vi "tb_Ping Pong BRAM.vi"() -> ()   [LabVIEW 2011]
panel:
  out "interleaved array":dbl[](array[numeric])
  out "Array 2":u16[](array[numeric])
  out "Array":u16[](array[numeric])
  out "Memory":u16[](array[numeric])
  in  "Iterations":i32=100
  out "Read Address":u16[](array[numeric])
  out "Output Data":u16[](array[numeric])
  in  "Write Count":u16
  in  "Read Count":u16
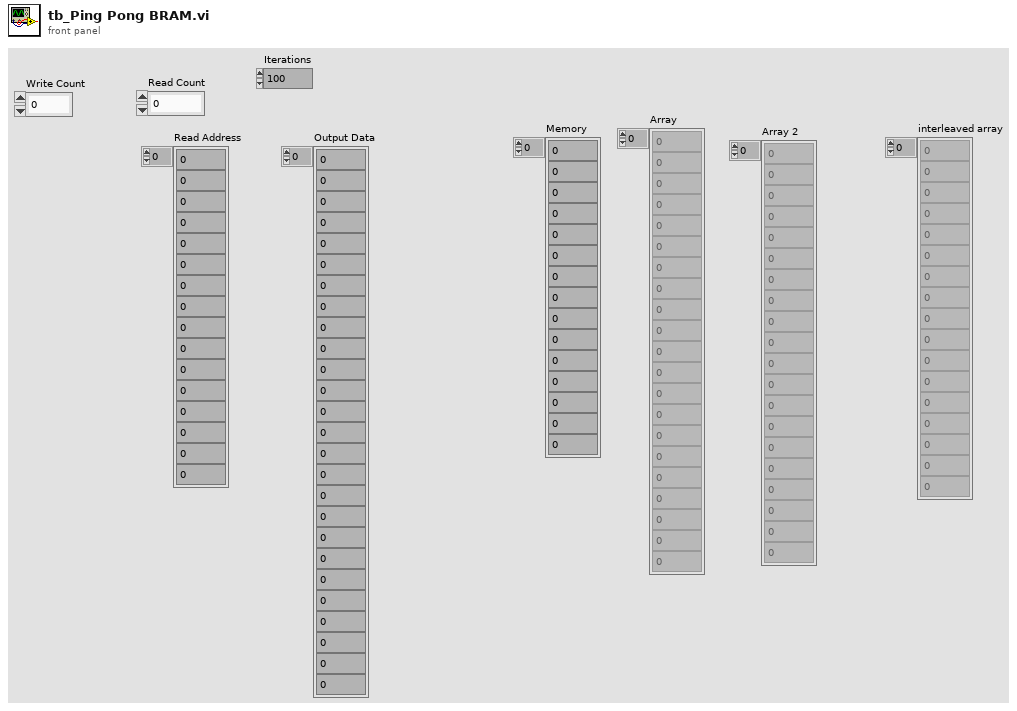
[diagram p1: front panel]
types:
  T1 = cluster{"Data 1":u16, "Data Valid 1":bool, "Address1":u16}
  T2 = cluster{"Data 2":u16, "Data Valid 2":bool, "Address 2":u16}
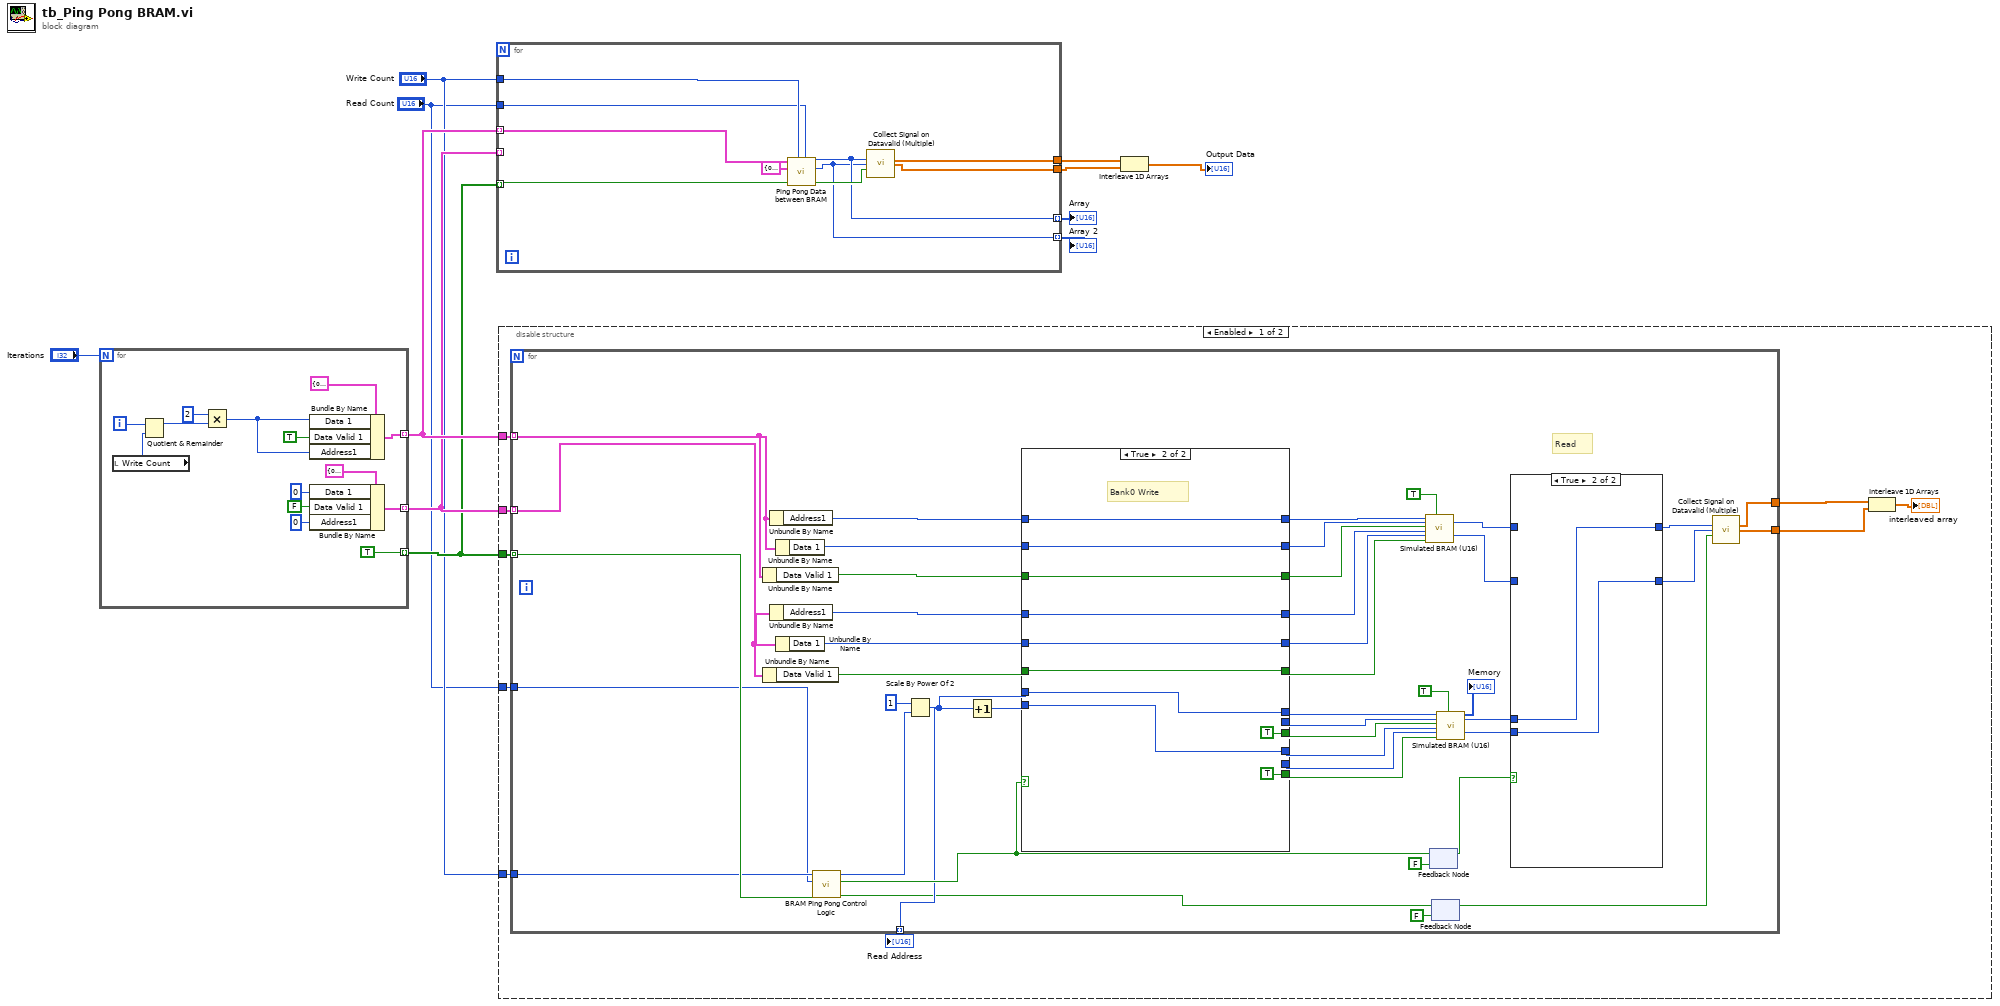
[diagram p0: block diagram]
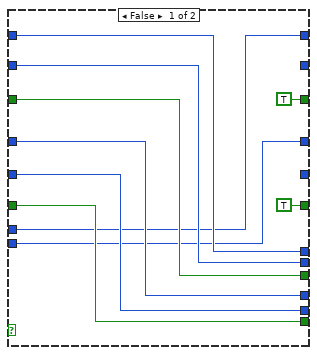
[diagram p3: hidden frame]
diagram:
  n1 = for {
    N: "Iterations" -> [_]
    tunnel: [w24] -> w10 mode=indexing
    tunnel: [w21] -> w9 mode=indexing
    tunnel: [TRUE] -> w8 mode=indexing
    i -> [w16]
    n2 = local read "Write Count"() -> (w14:u16)
    n3 = Quotient & Remainder(x=w16, y=w14) -> (x-y*floor(x/y)=w15:i32)  [unwired: 1 out]
    n4 = Multiply(x=2, y=w15) -> (x*y=w12:i32)
    n5 = Bundle By Name(cluster=T1 {"Data 1"=0, "Data Valid 1"=FALSE, "Address1"=0} ("Bank0 Data"), "Data 1"=w12, "Data Valid 1"=TRUE, "Address1"=w12) -> (w24:T1)
    n6 = Bundle By Name(cluster=T1 {"Data 1"=0, "Data Valid 1"=FALSE, "Address1"=0} ("Bank0 Data"), "Data 1"=u16 0, "Data Valid 1"=FALSE, "Address1"=u16 0) -> (w21:T1)
  }
  n7 = for {
    tunnel: w10 -> [w34] mode=indexing
    tunnel: w9 -> [_] mode=indexing
    tunnel: w8 -> [w35] mode=indexing
    tunnel: [w32] -> w7
    tunnel: [w31] -> w6
    tunnel: "Write Count" -> [w27]
    tunnel: "Read Count" -> [w26]
    tunnel: [w29] -> w2 mode=indexing
    tunnel: [w28] -> w1 mode=indexing
    n8 = call <userlib>:"Ping Pong Data between BRAM.vi"("Read Count"=w26, "Write Count"=w27, "Input Valid"=w35, "Bank1 Data"=T2 {"Data 2"=0, "Data Valid 2"=FALSE, "Address 2"=0}, "Bank0 Data"=w34) -> ("Read Valid"=w33:bool, "Address1. Element Out"=w28:u16, "Address0. Element Out"=w29:u16)  [unwired: 4 in]
    n9 = call <userlib>:"Collect Signal on Datavalid (Multiple).vi"("Input 1"=w29, "Input 2"=w28, "Data Valid"=w33) -> ("Output 1"=w32:dbl[], "Output 2"=w31:dbl[])  [unwired: 11 in]
  }
  "Array" <- w2
  "Array 2" <- w1
  n10 = disable-structure shown="Enabled" {
    disable-tunnel: w10 -> [w41 _]
    disable-tunnel: w9 -> [w40 _]
    disable-tunnel: w8 -> [w39 _]
    disable-tunnel: "Write Count" -> [w38 _]
    disable-tunnel: "Read Count" -> [w37 _]
    frame Enabled {
      n11 = for {
        tunnel: w41 -> [w88] mode=indexing
        tunnel: w40 -> [w87] mode=indexing
        tunnel: w39 -> [w86] mode=indexing
        tunnel: [w58] -> w44 mode=indexing
        tunnel: [w52] -> w43
        tunnel: [w51] -> w42
        tunnel: w38 -> [w46]
        tunnel: w37 -> [w45]
        # "Read"
        n12 = Unbundle By Name(w88) -> ("Data Valid 1"=w70:bool)
        n13 = Unbundle By Name(w87) -> ("Data Valid 1"=w76:bool)
        n14 = Unbundle By Name(w88) -> ("Address1"=w68:u16)
        n15 = Unbundle By Name(w87) -> ("Address1"=w72:u16)
        n16 = Unbundle By Name(w88) -> ("Data 1"=w67:u16)
        n17 = Unbundle By Name(w87) -> ("Data 1"=w73:u16)
        n18 = call <userlib>:"BRAM Ping Pong Control Logic.vi"("Input Valid"=w86, "Read Count"=w45, "Write Count"=w46) -> ("Read Valid"=w53:bool, "BRAM Bank0 Write?"=w60:bool, "Read Address"=w61:u16)  [unwired: 6 in]
        n19 = Scale By Power Of 2(n=1, x=w61) -> (x*2^n=w58:u16)
        n20 = Increment(x=w58) -> (x+1=w85:u16)
        n21 = case shown="True" w60 {
          tunnel: w67 -> [w101 w111]
          tunnel: w70 -> [w100 w110]
          tunnel: [_ w111] -> w62
          tunnel: w68 -> [w102 w112]
          tunnel: [w94 w112] -> w69
          tunnel: [TRUE ("Data Valid 1") w110] -> w71
          tunnel: w72 -> [w99 w109]
          tunnel: [w93 w109] -> w74
          tunnel: w73 -> [w98 w108]
          tunnel: [_ w108] -> w75
          tunnel: w76 -> [w97 w107]
          tunnel: [TRUE ("Data Valid 2") w107] -> w77
          tunnel: [w102 w104] -> w78
          tunnel: [w101 _] -> w79
          tunnel: [w100 TRUE ("Data Valid 1")] -> w80
          tunnel: [w99 w103] -> w81
          tunnel: [w98 _] -> w82
          tunnel: [w97 TRUE ("Data Valid 2")] -> w83
          tunnel: w58 -> [w94 w104]
          tunnel: w85 -> [w93 w103]
          frame False {
          }
          frame True {
            # "Bank0 Write"
          }
        }
        n22 = call <userlib>:"Simulated BRAM (U16).vi"("Address 0"=w69, "Address0.Element In"=w62, "Address 0 Write"=w71, "Address 1"=w74, "Address1.Element In"=w75, "Address 1 Write"=w77, "Read Before Write?"=TRUE) -> ("Address0. Element Out"=w63:u16, "Address1. Element Out"=w64:u16)  [unwired: 10 in, 1 out]
        n23 = feedback-in #1(w60) -> ()
        n24 = feedback #1(FALSE ("BRAM Bank0 Write?")) -> (w48:bool)
        n25 = feedback-in #2(w53) -> ()
        n26 = feedback #2(FALSE ("Read Valid")) -> (w50:bool)
        n27 = call <userlib>:"Simulated BRAM (U16).vi"("Address 0"=w78, "Address0.Element In"=w79, "Address 0 Write"=w80, "Address 1"=w81, "Address1.Element In"=w82, "Address 1 Write"=w83, "Read Before Write?"=TRUE) -> ("Memory"=→"Memory":u16[], "Address0. Element Out"=w65:u16, "Address1. Element Out"=w66:u16)  [unwired: 10 in]
        n28 = case shown="True" w48 {
          tunnel: w63 -> [w90 _]
          tunnel: w64 -> [w89 _]
          tunnel: w65 -> [_ w92]
          tunnel: w66 -> [_ w91]
          tunnel: [w90 w92] -> w55
          tunnel: [w89 w91] -> w54
          frame False {
          }
          frame True {
          }
        }
        n29 = call <userlib>:"Collect Signal on Datavalid (Multiple).vi"("Input 1"=w55, "Input 2"=w54, "Data Valid"=w50) -> ("Output 1"=w52:dbl[], "Output 2"=w51:dbl[])  [unwired: 11 in]
      }
      "Read Address" <- w44
      n30 = Interleave 1D Arrays(w43, w42) -> (→"interleaved array":dbl[])
    }
    frame Disabled {
    }
  }
  n31 = Interleave 1D Arrays(w7, w6) -> (→"Output Data":dbl[])
